vi "Sandbox3.vi"() -> ()   [LabVIEW 2014]
uses:
  <vilib>/xml/Load XML File.vi
  <vilib>/xml/Close Reference(Node).vi
  <vilib>/xml/Close Reference(NNMap).vi
  <vilib>/xml/NI_XML.lvlib
  <resource>/objmgr/DOMUserDefRef.rc
panel:
  out "Values":string[][](array[string])
  out "Names":string[][](array[string])
  in  "path to XML document":path
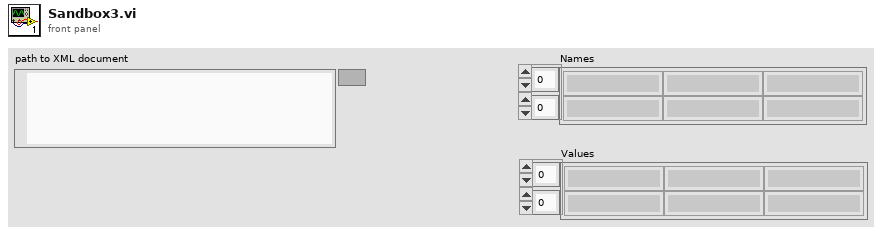
[diagram p1: front panel]
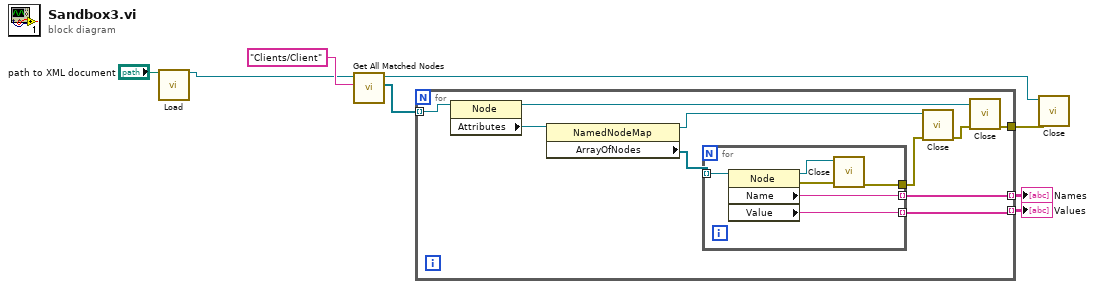
[diagram p0: block diagram]
diagram:
  n1 = call-poly <vilib>:"Load.vi"("path to XML document"="path to XML document") -> ("DOM document out"=w6:refnum<k20>)  [unwired: 12 in, 2 out]
  n2 = call <vilib>:"Get All Matched Nodes.vi"("XPath expression"="Clients/Client", "node in"=w6) -> ("node result array"=w5:refnum<k20>[], "node out"=w1:refnum<k20>)  [unwired: 7 in, 1 out]
  n3 = for {
    tunnel: w5 -> [w18] mode=indexing
    tunnel: [w15] -> w4 mode=indexing
    tunnel: [w14] -> w3 mode=indexing
    tunnel: [w9] -> w2
    n4 = property class="Node"(reference=w18) -> (reference out=w10:refnum<k20>, "Attributes"=w17:refnum<k20>)  [unwired: 1 in, 1 out]
    n5 = property class="NamedNodeMap"(reference=w17) -> (reference out=w12:refnum<k20>, "ArrayOfNodes"=w16:refnum<k20>[])  [unwired: 1 in, 1 out]
    n6 = for {
      tunnel: w16 -> [w24] mode=indexing
      tunnel: [w23] -> w15 mode=indexing
      tunnel: [w22] -> w14 mode=indexing
      tunnel: [w19] -> w13
      n7 = property class="Node"(reference=w24) -> (reference out=w20:refnum<k20>, error out=w21:errorcluster, "Name"=w23:string, "Value"=w22:string)  [unwired: 1 in]
      n8 = call-poly <vilib>:"Close.vi"("error in (no error)"=w21, "node"=w20) -> ("error out"=w19:errorcluster)  [unwired: 7 in]
    }
    n9 = call-poly <vilib>:"Close.vi"("error in (no error)"=w13, "named node map"=w12) -> ("error out"=w11:errorcluster)  [unwired: 7 in]
    n10 = call-poly <vilib>:"Close.vi"("error in (no error)"=w11, "node"=w10) -> ("error out"=w9:errorcluster)  [unwired: 7 in]
  }
  "Names" <- w4
  "Values" <- w3
  n11 = call-poly <vilib>:"Close.vi"("error in (no error)"=w2, "node"=w1) -> ()  [unwired: 7 in, 1 out]
